vi "DT_Dependencies_CSS_JS.vi"() -> (1 "DT_Extensions_JS_Files":path[](array[path]), 2 "DT_Extensions_CSS_Files":path[](array[path]))   [LabVIEW 2014]
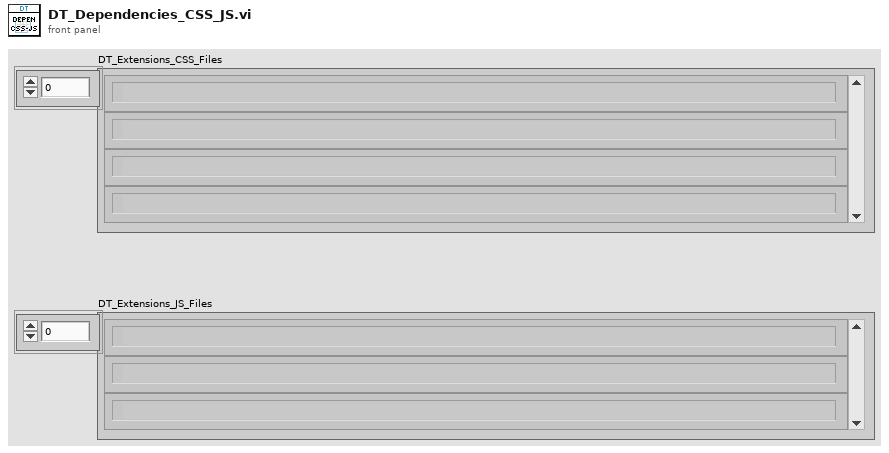
[diagram p1: front panel]
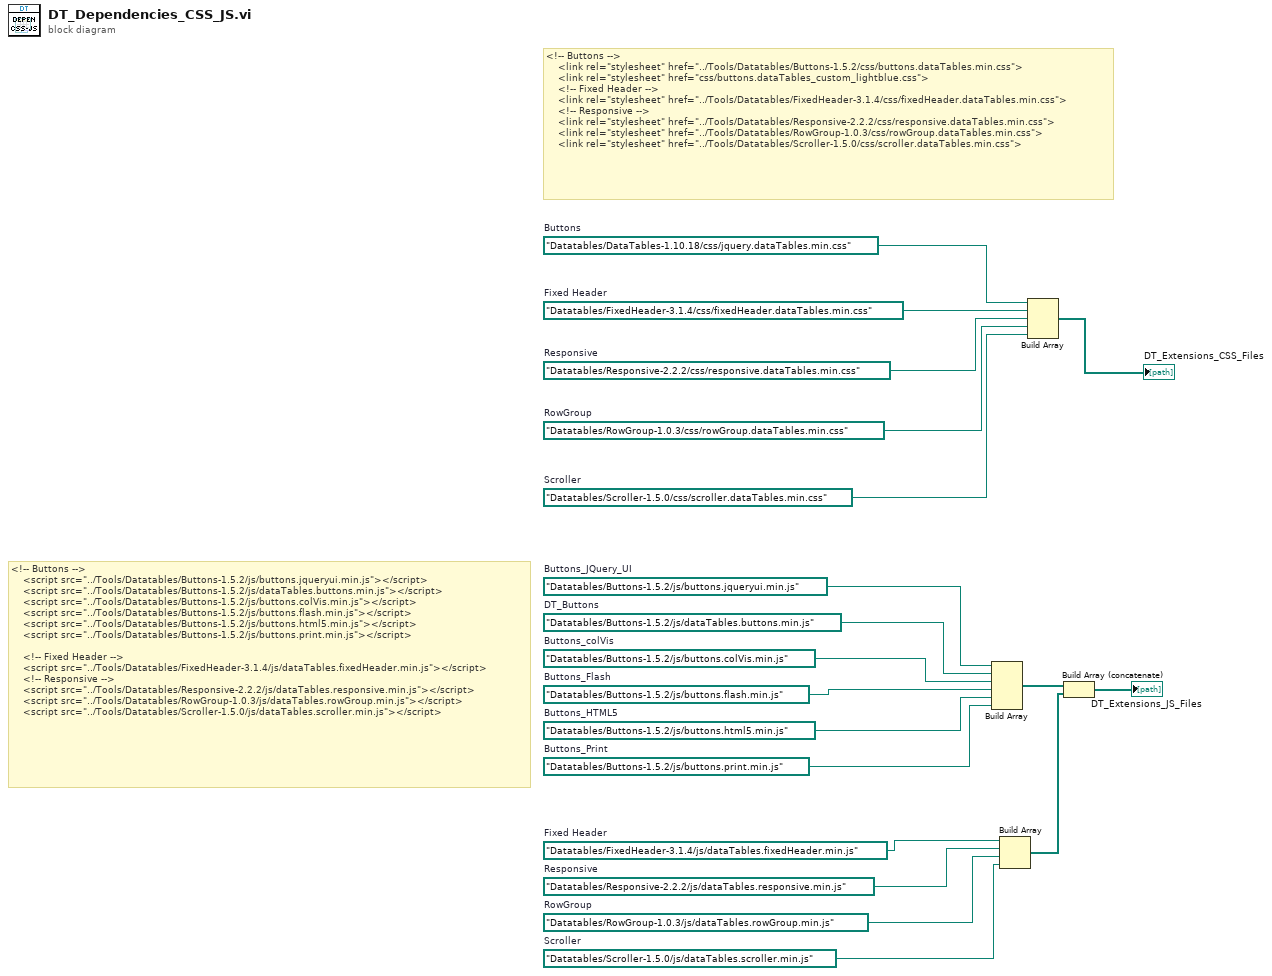
[diagram p0: block diagram]
diagram:
  w2 = path "Datatables/Scroller-1.5.0/js/dataTables.scroller.min.js"  # Scroller
  w3 = path "Datatables/RowGroup-1.0.3/js/dataTables.rowGroup.min.js"  # RowGroup
  w4 = path "Datatables/Responsive-2.2.2/js/dataTables.responsive.min.js"  # Responsive
  w5 = path "Datatables/FixedHeader-3.1.4/js/dataTables.fixedHeader.min.js"  # Fixed Header
  w8 = path "Datatables/Buttons-1.5.2/js/buttons.print.min.js"  # Buttons_Print
  w13 = path "Datatables/Buttons-1.5.2/js/buttons.html5.min.js"  # Buttons_HTML5
  w12 = path "Datatables/Buttons-1.5.2/js/buttons.flash.min.js"  # Buttons_Flash
  w11 = path "Datatables/Buttons-1.5.2/js/buttons.colVis.min.js"  # Buttons_colVis
  w10 = path "Datatables/Buttons-1.5.2/js/dataTables.buttons.min.js"  # DT_Buttons
  w9 = path "Datatables/Buttons-1.5.2/js/buttons.jqueryui.min.js"  # Buttons_JQuery_UI
  w14 = path "Datatables/Scroller-1.5.0/css/scroller.dataTables.min.css"  # Scroller
  w15 = path "Datatables/RowGroup-1.0.3/css/rowGroup.dataTables.min.css"  # RowGroup
  w16 = path "Datatables/Responsive-2.2.2/css/responsive.dataTables.min.css"  # Responsive
  w17 = path "Datatables/FixedHeader-3.1.4/css/fixedHeader.dataTables.min.css"  # Fixed Header
  w19 = path "Datatables/DataTables-1.10.18/css/jquery.dataTables.min.css"  # Buttons
  # "<!-- Buttons -->\n    <script src=\"../Tools/Datatables/Buttons-1.5.2/js/buttons.jqueryui.min.js\"></script>\n    <script src=\"../Tools/Datatables/Buttons-1.5.2/js/dataTables.buttons.min.js\"></script>\n    <script src=\"../Tools/Datatables/Buttons-1.5.2/js/buttons.colVis.min.js\"></script>\n    <script src=\"../Tools/Datatables/Buttons-1.5.2/js/buttons.flash.min.js\"></script>\n    <script src=\"../Tools/Datatables/Buttons-1.5.2/js/buttons.html5.min.js\"></script>\n    <script src=\"../Tools/Datatables/Buttons-1.5.2/js/buttons.print.min.js\"></script>\n    \n    <!-- Fixed Header -->\n    <script src=\"../Tools/Datatables/FixedHeader-3.1.4/js/dataTables.fixedHeader.min.js\"></script>\n    <!-- Responsive -->\n    <script src=\"../Tools/Datatables/Responsive-2.2.2/js/dataTables.responsive.min.js\"></script>\n    <script src=\"../Tools/Datatables/RowGroup-1.0.3/js/dataTables.rowGroup.min.js\"></script>\n    <script src=\"../Tools/Datatables/Scroller-1.5.0/js/dataTables.scroller.min.js\"></script>"
  # "<!-- Buttons -->\n    <link rel=\"stylesheet\" href=\"../Tools/Datatables/Buttons-1.5.2/css/buttons.dataTables.min.css\">\n    <link rel=\"stylesheet\" href=\"css/buttons.dataTables_custom_lightblue.css\">\n    <!-- Fixed Header -->\n    <link rel=\"stylesheet\" href=\"../Tools/Datatables/FixedHeader-3.1.4/css/fixedHeader.dataTables.min.css\">\n    <!-- Responsive -->\n    <link rel=\"stylesheet\" href=\"../Tools/Datatables/Responsive-2.2.2/css/responsive.dataTables.min.css\">\n    <link rel=\"stylesheet\" href=\"../Tools/Datatables/RowGroup-1.0.3/css/rowGroup.dataTables.min.css\">\n    <link rel=\"stylesheet\" href=\"../Tools/Datatables/Scroller-1.5.0/css/scroller.dataTables.min.css\">"
  n1 = Build Array(w9, w10, w11, w12, w13, w8) -> (w7:path[])
  n2 = Build Array(w5, w4, w3, w2) -> (w1:path[])
  n3 = Build Array(w19, w17, w16, w15, w14) -> (→"DT_Extensions_CSS_Files":path[])
  n4 = Build Array (concatenate)(w7, w1) -> (→"DT_Extensions_JS_Files":path[])
